vi "Post-Project-Copying Process - Stage 2.vi"(8 "error in":errorcluster, 11 "PluginGenerator_MetaDataObj":refnum<class "PluginGenerator_MetaDataObj.lvclass">) -> (0 "error out":errorcluster, 3 "PluginGenerator_MetaDataObj out":refnum<class "PluginGenerator_MetaDataObj.lvclass">)   [LabVIEW 2023, in "Plugin Generator.lvlib"]
uses:
  Plugin Generator.lvlib
  PluginGenerator_MetaDataObj/PluginGenerator_MetaDataObj.lvclass
  c:/perforce/build/exports/ni/nito/nitoolchainlabview2023eng64/official/export/23.3/23.3.0f52/win/resource/dialog/NewProjectWizard/MetaDataObj/MetaDataObj.lvclass
  <resource>/dialog/NewProjectWizard/MetaDataObj/MetaDataObj.lvclass/MetaDataObj.ctl
  <resource>/dialog/NewProjectWizard/MetaDataObj/Accessors/Read Project Name.vi
  <vilib>/dlg_ctls.llb/Space Constant.vi
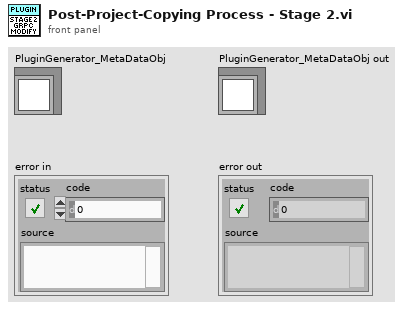
[diagram p1: front panel]
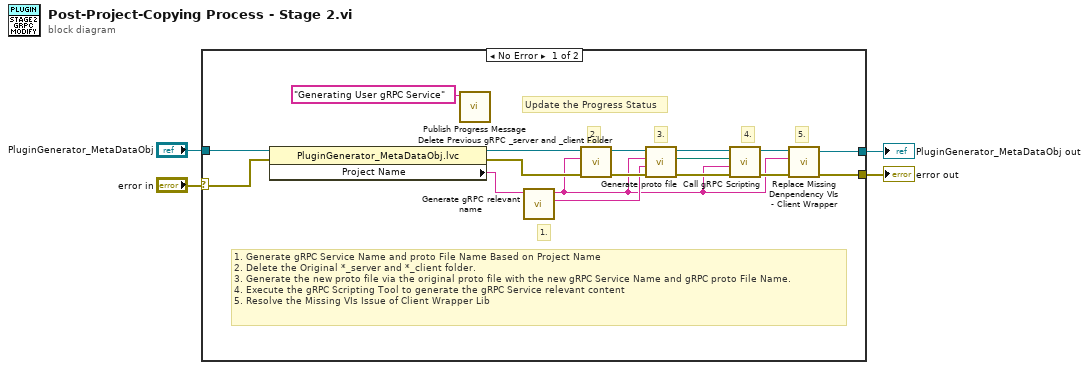
[diagram p0: block diagram]
diagram:
  n1 = case shown="No Error" "error in" {
    selector: "error in" -> [w5 w23]
    tunnel: [w21 w23] -> w4
    tunnel: "PluginGenerator_MetaDataObj" -> [w20 w22]
    tunnel: [w7 w22] -> w2
    frame No Error {
      # "5."
      # "4."
      # "3."
      # "2."
      # "1."
      # "1. Generate gRPC Service Name and proto File Name Based on Project Name\n2. Delete the Original *_server and *_client folder.\n3. Generate the new proto file via the original proto file with the new gRPC Service Name and gRPC proto File Name.\n4. Execute the gRPC Scripting Tool to generate the gRPC Service relevant content\n5. Resolve the Missing VIs Issue of Client Wrapper Lib"
      # "Update the Progress Status"
      n2 = property class="PluginGenerator_MetaDataObj.lvc"(reference=w20, error in=w5) -> (reference out=w15:refnum<class "PluginGenerator_MetaDataObj.lvclass">, error out=w18:errorcluster, "Project Name"=w10:string)
      n3 = call "Publish Progress Message.vi"("Progress"="Generating User gRPC Service") -> ()  [unwired: 11 in]
      n4 = call "Generate gRPC relevant name.vi"("Project Name"=w10) -> ("gRPC proto File Name"=w9:string, "gRPC Service Name"=w8:string)  [unwired: 9 in]
      n5 = call "Delete Previous gRPC _server and _client Folder.vi"("error in"=w18, "gRPC Service Name"=w8, "PluginGenerator_MetaDataObj"=w15) -> ("error out"=w19:errorcluster, "PluginGenerator_MetaDataObj out"=w14:refnum<class "PluginGenerator_MetaDataObj.lvclass">)  [unwired: 7 in]
      n6 = call "Generate proto file.vi"("error in"=w19, "gRPC proto File Name"=w9, "gRPC Service Name"=w8, "PluginGenerator_MetaDataObj"=w14) -> ("error out"=w17:errorcluster, "proto File Path"=w13:path, "PluginGenerator_MetaDataObj out"=w12:refnum<class "PluginGenerator_MetaDataObj.lvclass">)  [unwired: 5 in]
      n7 = call "Call gRPC Scripting.vi"("error in"=w17, "gRPC Service Name"=w8, "proto File Path"=w13, "PluginGenerator_MetaDataObj"=w12) -> ("error out"=w16:errorcluster, "PluginGenerator_MetaDataObj out"=w11:refnum<class "PluginGenerator_MetaDataObj.lvclass">)  [unwired: 6 in]
      n8 = call "Replace Missing Denpendency VIs - Client Wrapper.vi"("error in"=w16, "gRPC Service Name"=w8, "PluginGenerator_MetaDataObj"=w11) -> ("error out"=w21:errorcluster, "PluginGenerator_MetaDataObj out"=w7:refnum<class "PluginGenerator_MetaDataObj.lvclass">)  [unwired: 7 in]
    }
    frame Error {
    }
  }
  "error out" <- w4
  "PluginGenerator_MetaDataObj out" <- w2
